vi "LastScanFailedRed.vi"(8 "error in (no error)":errorcluster) -> (0 "error out":errorcluster)   [LabVIEW 2013]
panel:
  # "Last scan failed"
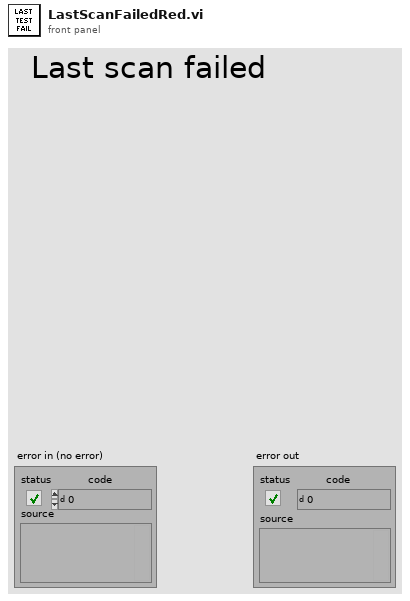
[diagram p1: front panel]
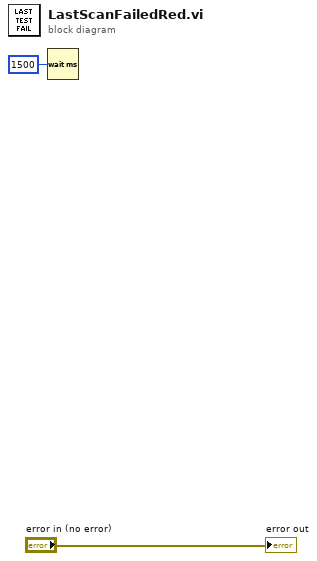
[diagram p0: block diagram]
diagram:
  n1 = Wait (ms)(milliseconds to wait=u32 1500) -> ()  [unwired: 1 out]
  "error out" <- "error in (no error)"
